vi "Move.vi"(5 "Force":bool=TRUE, 7 "Valve":string, 10 "max time":i32, 11 "Volcano in":refnum<class "Volcano.lvclass">) -> (1 "Finished?":bool, 2 "# elements in queue":i32, 3 "Volcano out":refnum<class "Volcano.lvclass">)   [LabVIEW 2021, in "d16.lvlib" / "Volcano.lvclass"]
uses:
  Volcano.lvclass
  Volcano.lvclass/Volcano.ctl
  <vilib>/Utility/miscctls.llb/LVMapReplaceAction.ctl
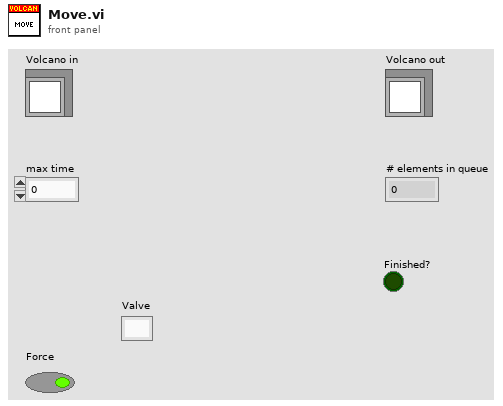
[diagram p1: front panel]
types:
  T1 = typedef "LVMapReplaceAction.ctl" = enum32{"Modify Entry only if found", "Add or Modify Entry", "Delete Entry"}
  T2 = cluster{"Current Valve":string, "Unopened Valves":string[], "Cumulative Pressure Released":u64, "Time":i32}
  T3 = map{string, cluster{"Flow Rate":i32, "Routes":string[], "Route Time":i32[]}}
  T4 = cluster{"Flow Rate":i32, "Routes":string[], "Route Time":i32[]}
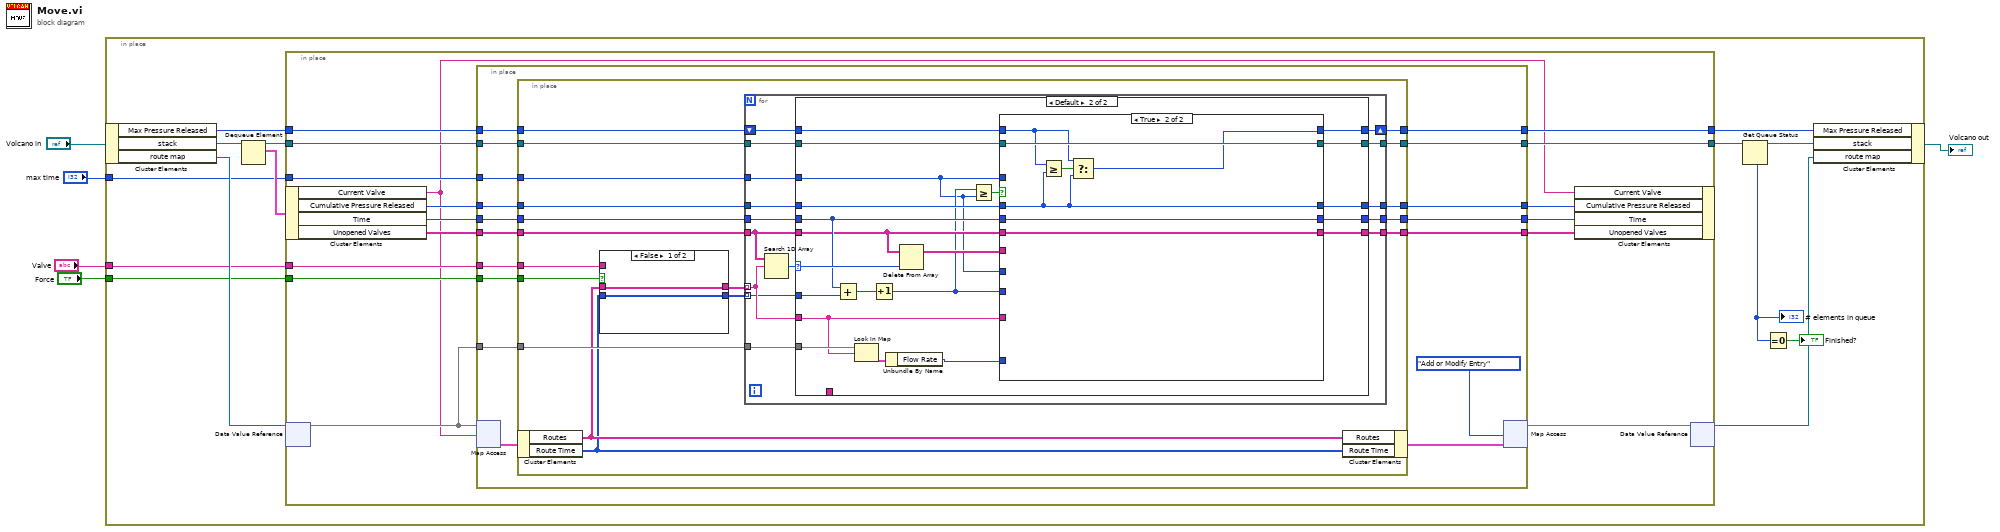
[diagram p0: block diagram]
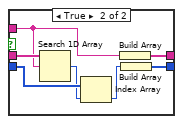
[diagram p2: hidden frame]
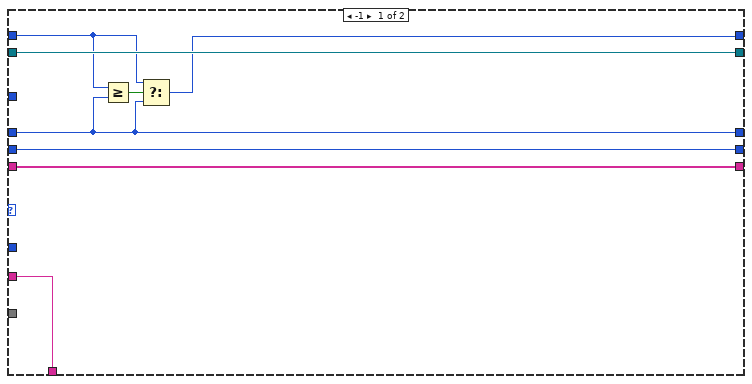
[diagram p3: hidden frame]
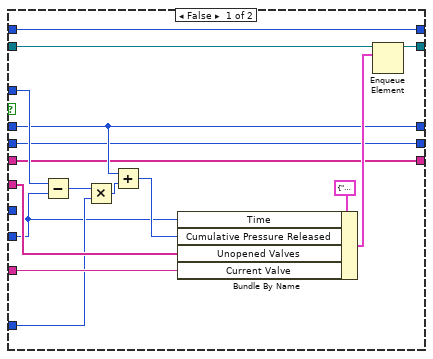
[diagram p4: hidden frame]
diagram:
  n1 = in-place {
    in-place-border: "max time" -> [w15]
    in-place-border: "Force" -> [w7]
    in-place-border: "Valve" -> [w6]
    n2 = in-place-cluster #1("Volcano in") -> ("Max Pressure Released"=w13:u64, "stack"=w19:refnum<queue>, "route map"=w17:refnum<data-value>)
    n3 = Dequeue Element(queue=w19) -> (queue out=w18:refnum<queue>, element=w16:T2)  [unwired: 2 in, 2 out]
    n4 = in-place {
      in-place-border: w18 -> [w35]
      in-place-border: w15 -> [w34]
      in-place-border: [w33] -> w11
      in-place-border: w13 -> [w31]
      in-place-border: [w30] -> w12
      in-place-border: w7 -> [w28]
      in-place-border: w6 -> [w27]
      n5 = in-place-cluster #2(w16) -> ("Current Valve"=w20:string, "Cumulative Pressure Released"=w24:u64, "Time"=w22:i32, "Unopened Valves"=w25:string[])
      n6 = in-place-dvr #3(w17) -> (w29:T3)  [unwired: 1 out]
      n7 = in-place {
        in-place-border: w35 -> [w50]
        in-place-border: w24 -> [w51]
        in-place-border: w34 -> [w44]
        in-place-border: [w49] -> w33
        in-place-border: w22 -> [w45]
        in-place-border: w31 -> [w43]
        in-place-border: [w42] -> w30
        in-place-border: w25 -> [w46]
        in-place-border: w29 -> [w41]
        in-place-border: w28 -> [w40]
        in-place-border: w27 -> [w39]
        in-place-border: [w38] -> w26
        in-place-border: [w37] -> w21
        in-place-border: [w36] -> w23
        n8 = in-place-map #4(w29, w20) -> (w52:T4)  [unwired: 1 in, 1 out]
        n9 = in-place {
          in-place-border: w45 -> [w66]
          in-place-border: w44 -> [w64]
          in-place-border: w51 -> [w65]
          in-place-border: w50 -> [w70]
          in-place-border: [w69] -> w49
          in-place-border: w46 -> [w67]
          in-place-border: w43 -> [w68]
          in-place-border: [w63] -> w42
          in-place-border: w41 -> [w62]
          in-place-border: w40 -> [w61]
          in-place-border: w39 -> [w56]
          in-place-border: [w55] -> w38
          in-place-border: [w54] -> w37
          in-place-border: [w53] -> w36
          n10 = in-place-cluster #5(w52) -> ("Routes"=w60:string[], "Route Time"=w59:i32[])
          n11 = case shown="False" w61 {
            tunnel: w60 -> [w72 w78]
            tunnel: w59 -> [w71 w76]
            tunnel: [w72 w79] -> w58
            tunnel: [w71 w73] -> w57
            tunnel: w56 -> [_ w77]
            frame False {
            }
            frame True {
              n12 = Search 1D Array(1D array=w78, element=w77) -> (index of element=w75:i32)  [unwired: 1 in]
              n13 = Index Array(array=w76, index=w75) -> (element=w74:i32)
              n14 = Build Array(w77) -> (w79:string[])
              n15 = Build Array(w74) -> (w73:i32[])
            }
          }
          n16 = for {
            tunnel: w70 -> [w94]
            tunnel: [w93] -> w69
            tunnel: w67 -> [w92]
            tunnel: w66 -> [w90]
            tunnel: w65 -> [w87]
            tunnel: w64 -> [w88]
            shift-right: [w86] -> w63
            shift-left: w68 -> [w89]
            tunnel: w62 -> [w85]
            tunnel: w58 -> [w84] mode=indexing
            tunnel: w57 -> [w83] mode=indexing
            tunnel: [w82] -> w55
            tunnel: [w81] -> w54
            tunnel: [w80] -> w53
            n17 = Search 1D Array(1D array=w92, element=w84) -> (index of element=w91:i32)  [unwired: 1 in]
            n18 = case shown="Default" w91 {
              selector: w91 -> [_ w121]
              tunnel: w94 -> [w102 w123]
              tunnel: [w102 w122] -> w93
              tunnel: w92 -> [w96 w107]
              tunnel: w90 -> [w97 w109]
              tunnel: w83 -> [_ w119]
              tunnel: w89 -> [w100 w117]
              tunnel: w88 -> [_ w103]
              tunnel: w87 -> [w98 w116]
              tunnel: [w101 w115] -> w86
              tunnel: w85 -> [_ w114]
              tunnel: w84 -> [w95 w113]
              tunnel: [w96 w106] -> w82
              tunnel: [w97 w108] -> w81
              tunnel: [w98 w110] -> w80
              tunnel: [w95 _] -> _
              frame -1 {
                n19 = Greater Or Equal?(x=w100, y=w98) -> (x >= y?=w99:bool)
                n20 = Select(t=w100, s=w99, f=w98) -> (s? t:f=w101:u64)
              }
              frame Default {
                n21 = Add(x=w109, y=w119) -> (x+y=w105:i32)
                n22 = Look In Map(map=w114, key=w113) -> (value=w112:T4)  [unwired: 1 in, 1 out]
                n23 = Increment(x=w105) -> (x+1=w104:i32)
                n24 = Unbundle By Name(w112) -> ("Flow Rate"=w111:i32)
                n25 = Delete From Array(array=w107, index=w121) -> (array with subset deleted=w120:string[])  [unwired: 1 in, 1 out]
                n26 = Greater Or Equal?(x=w104, y=w103) -> (x >= y?=w118:bool)
                n27 = case shown="True" w118 {
                  tunnel: w123 -> [w139 w146]
                  tunnel: [w137 w146] -> w122
                  tunnel: w120 -> [w134 _]
                  tunnel: w113 -> [w135 _]
                  tunnel: w117 -> [w128 w145]
                  tunnel: w111 -> [w132 _]
                  tunnel: w104 -> [w126 _]
                  tunnel: w103 -> [w131 _]
                  tunnel: w116 -> [w127 w140]
                  tunnel: [w128 w144] -> w115
                  tunnel: [w127 w140] -> w110
                  tunnel: w107 -> [w124 w142]
                  tunnel: w109 -> [w125 w143]
                  tunnel: [w125 w143] -> w108
                  tunnel: [w124 w142] -> w106
                  tunnel: w103 -> [_ _]
                  frame False {
                    n28 = Subtract(x=w131, y=w126) -> (x-y=w133:i32)
                    n29 = Multiply(x=w133, y=w132) -> (x*y=w130:i32)
                    n30 = Add(x=w127, y=w130) -> (x+y=w129:u64)
                    n31 = Bundle By Name(cluster=T2 {"Current Valve"="", "Unopened Valves"=[], "Cumulative Pressure Released"=0, "Time"=0} ("element"), "Time"=w126, "Cumulative Pressure Released"=w129, "Unopened Valves"=w134, "Current Valve"=w135) -> (w138:T2)
                    n32 = Enqueue Element(queue=w139, element=w138) -> (queue out=w137:refnum<queue>)  [unwired: 2 in, 2 out]
                  }
                  frame True {
                    n33 = Greater Or Equal?(x=w145, y=w140) -> (x >= y?=w141:bool)
                    n34 = Select(t=w145, s=w141, f=w140) -> (s? t:f=w144:u64)
                  }
                }
              }
            }
          }
          n35 = in-place-cluster #5("Routes"=w60, "Route Time"=w59) -> (w48:T4)
        }
        n36 = in-place-map #4(w48, LVMapReplaceAction."Add or Modify Entry" ("action")) -> (w32:T3)  [unwired: 2 out]
      }
      n37 = in-place-cluster #2("Current Valve"=w20, "Cumulative Pressure Released"=w23, "Time"=w21, "Unopened Valves"=w26) -> ()  [unwired: 1 out]
      n38 = in-place-dvr #3(w32) -> (w14:refnum<data-value>)  [unwired: 1 out]
    }
    n39 = Get Queue Status(queue=w11) -> (queue out=w10:refnum<queue>, # elements in queue=w9:i32)  [unwired: 2 in, 6 out]
    "# elements in queue" <- w9
    n40 = Equal To 0?(x=w9) -> (x = 0?=→"Finished?":bool)
    n41 = in-place-cluster #1("Max Pressure Released"=w12, "stack"=w10, "route map"=w14) -> (→"Volcano out":refnum<class "Volcano.lvclass">)
  }
